vi "Excel_Title.vi"(7 "Report_Title":T1, 8 "error in (no error)":errorcluster, 10 "Report path in":path, 11 "Template path":path) -> (0 "error out":errorcluster, 2 "Report path out":path, 3 "report out":refnum<class "NI_report.lvclass">)   [LabVIEW 2015]
doc: "报表右上角的一大坨\n从编号到载荷时间"
uses:
  CustomControl/ReportTitle.ctl
  <vilib>/Utility/NIReport.llb/NI_report.lvclass
  <vilib>/addons/_office/NI_ReportGenerationToolkit.lvlib
  CustomControl/EnumReportTitle.ctl
panel:
  out "errorout":errorcluster
  in  "start(-1,-1) 2":cluster{"row":i32, "column":i32}
  in  "start(-1,-1)":cluster{"row":i32, "column":i32}
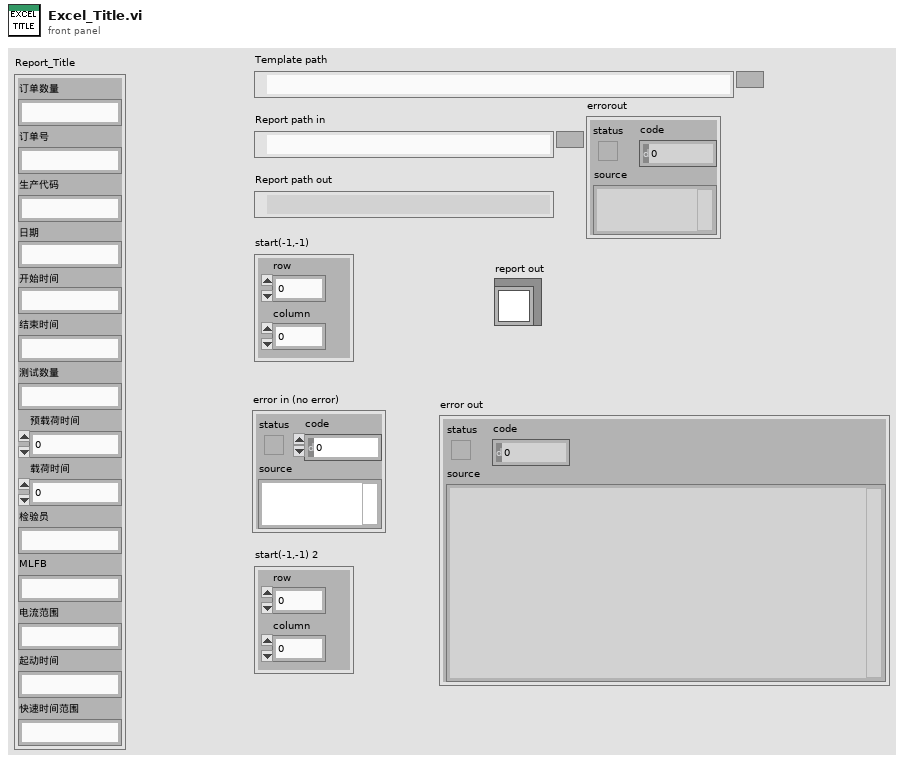
[diagram p1: front panel]
types:
  T1 = typedef "ReportTitle.ctl" = cluster{"订单数量":string, "订单号":string, "生产代码":string, "日期":string, "开始时间":string, "结束时间":string, "测试数量":string, "预载荷时间":i32, "载荷时间":i32, "检验员":string, "MLFB":string, "电流范围":string, "起动时间":string, "快速时间范围":string}
  T2 = enum16{"Standard Report", "HTML", "Word", "Excel"}
  T3 = enum16{"maximized", "minimized", "normal", "no change"}
  T4 = typedef "EnumReportTitle.ctl" = enum16{"CreatNewReport", "编号", "MLFB", "电流范围", "订单号", "订单数量", "测试日期", "检验员", "生产代码", "测试开始", "测试结束", "测试数量", "预载荷时间", "载荷时间", "起动时间", "快速动作范围", "CloseReport"}
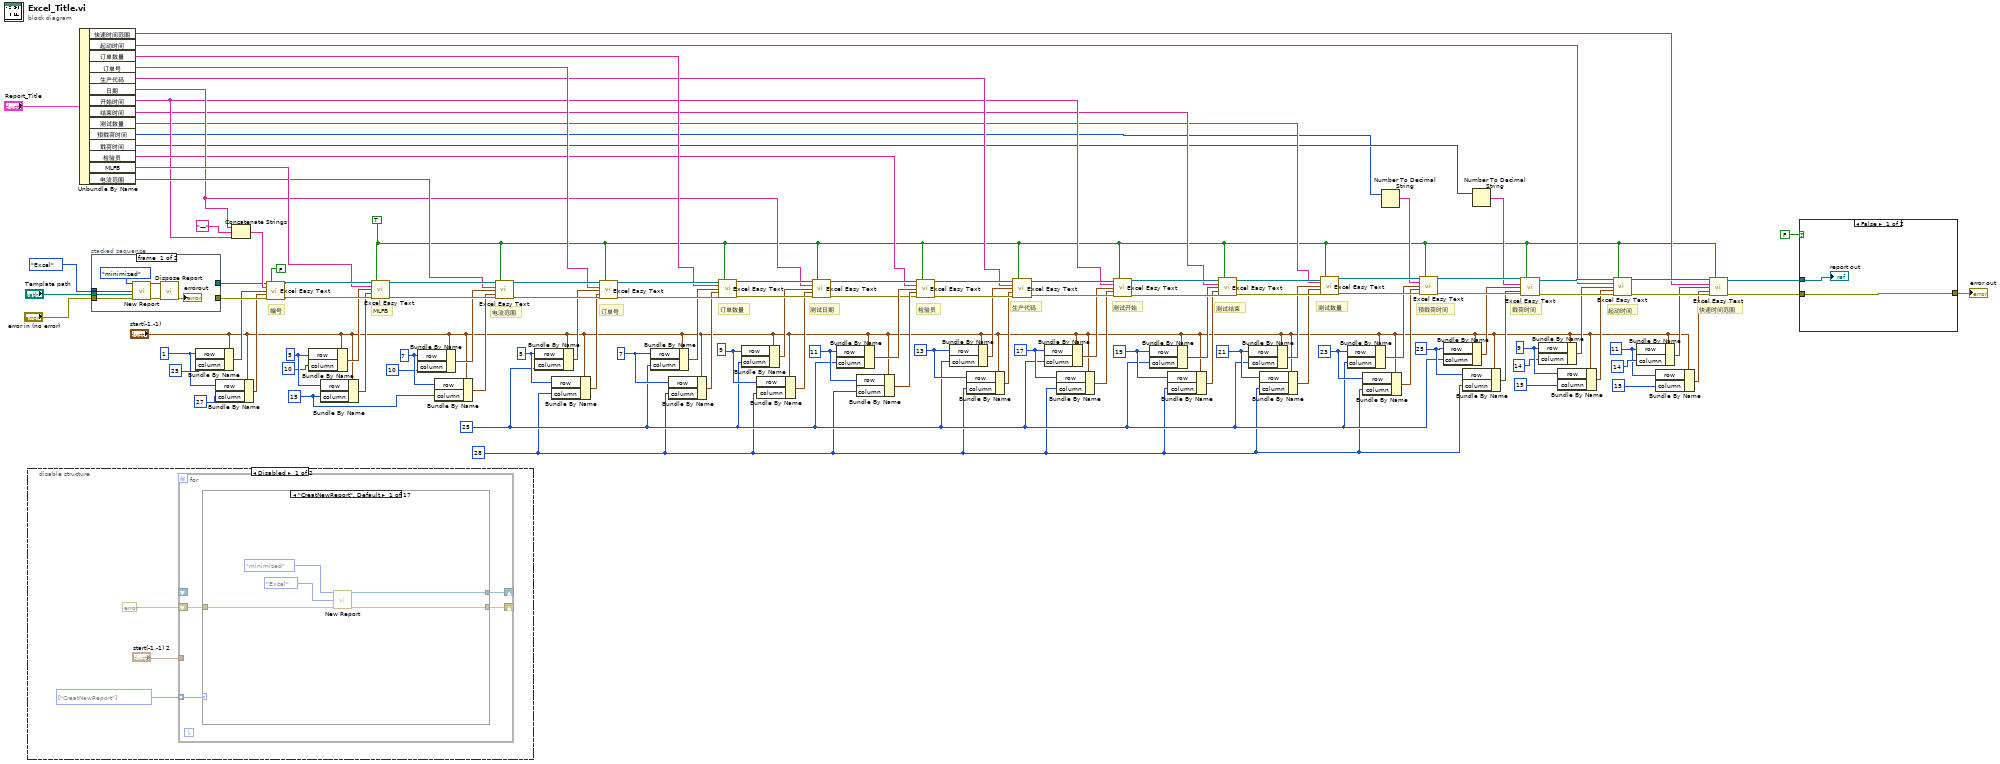
[diagram p0: block diagram]
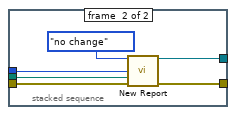
[diagram p2: hidden frame]
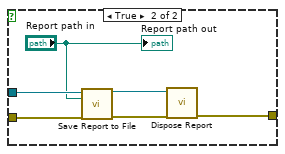
[diagram p20: hidden frame]
diagram:
  w5 = 11 ("row")
  w10 = 9 ("row")
  w43 = 25 ("row")
  w48 = 23 ("row")
  w53 = 21 ("row")
  w58 = 19 ("row")
  w63 = 17 ("row")
  w68 = 13 ("row")
  w75 = 11 ("row")
  w80 = 9 ("row")
  w41 = 28 ("column")
  w42 = 25 ("column")
  w83 = 7 ("column")
  w90 = 5 ("row")
  w103 = 7 ("row")
  w95 = 15 ("column")
  w99 = 5 ("row")
  w13 = TRUE ("border? (F)")
  w109 = 1 ("row")
  # "快速时间范围"
  # "起动时间"
  # "载荷时间"
  # "预载荷时间"
  # "测试数量"
  # "测试结束"
  # "测试开始"
  # "生产代码"
  # "检验员"
  # "测试日期"
  # "订单数量"
  # "订单号"
  # "编号"
  # "电流范围"
  # "MLFB"
  n1 = disable-structure shown="Disabled" {
    frame Disabled {
      w118 = T4[] [enum."CreatNewReport"] items=["CreatNewReport", "编号", "MLFB", "电流范围", "订单号", "订单数量", "测试日期", "检验员", "生产代码", "测试开始", "测试结束", "测试数量", "预载荷时间", "载荷时间", "起动时间", "快速动作范围", "CloseReport"]
      n2 = for {
        tunnel: w118 -> [w122] mode=indexing
        shift-right: [w120] -> _
        shift-left: errorcluster {"status"=FALSE, "code"=0, "source"=""} ("error out") -> [w121]
        shift-right: [w119] -> _
        shift-left: _ -> [_]
        tunnel: "start(-1,-1) 2" -> [_]
        n3 = case shown="\"CreatNewReport\", Default" w122 {
          tunnel: w121 -> [w125 _ _ _ _ _ _ _ _ _ _ _ _ _ _ _ _]
          tunnel: [w124 _ _ _ _ _ _ _ _ _ _ _ _ _ _ _ _] -> w120
          tunnel: [w123 _ _ _ _ _ _ _ _ _ _ _ _ _ _ _ _] -> w119
          frame "CreatNewReport", Default {
            n4 = call <vilib>:"New Report.vi"("window state (normal)"=T3."minimized", "report type"=T2."Excel", "error in (no error)"=w125) -> ("report out"=w123:refnum<class "NI_report.lvclass">, "error out"=w124:errorcluster)  [unwired: 11 in]
          }
          frame "编号" {
          }
          frame "MLFB" {
          }
          frame "电流范围" {
          }
          frame "订单号" {
          }
          frame "订单数量" {
          }
          frame "测试日期" {
          }
          frame "检验员" {
          }
          frame "生产代码" {
          }
          frame "测试开始" {
          }
          frame "测试结束" {
          }
          frame "测试数量" {
          }
          frame "预载荷时间" {
          }
          frame "载荷时间" {
          }
          frame "起动时间" {
          }
          frame "快速动作范围" {
          }
          frame "CloseReport" {
          }
        }
      }
    }
    frame Enabled {
    }
  }
  n5 = Unbundle By Name("Report_Title") -> ("快速时间范围"=w14:string, "起动时间"=w17:string, "订单数量"=w35:string, "订单号"=w36:string, "生产代码"=w32:string, "日期"=w34:string, "开始时间"=w31:string, "结束时间"=w30:string, "测试数量"=w29:string, "预载荷时间"=w25:i32, "载荷时间"=w27:i32, "检验员"=w33:string, "MLFB"=w38:string, "电流范围"=w37:string)
  n6 = stacked-sequence {
    tunnel: T2."Excel" ("report type") -> [w134 w138]
    tunnel: "Template path" -> [w133 w137]
    tunnel: "error in (no error)" -> [w132 w136]
    tunnel: [_ w140] -> w113
    tunnel: [_ w139] -> w114
    frame #0 {
      n7 = call <vilib>:"New Report.vi"("window state (normal)"=T3."minimized", "report type"=w134, "template (empty)"=w133, "error in (no error)"=w132) -> ("report out"=w130:refnum<class "NI_report.lvclass">, "error out"=w131:errorcluster)  [unwired: 10 in]
      n8 = call-dynamic "Dispose Report.vi"("report in"=w130, "error in (no error)"=w131) -> ("error out"=→"errorout":errorcluster)  [unwired: 13 in]
    }
    frame #1 {
      n9 = call <vilib>:"New Report.vi"("window state (normal)"=T3."no change", "report type"=w138, "template (empty)"=w137, "error in (no error)"=w136) -> ("report out"=w139:refnum<class "NI_report.lvclass">, "error out"=w140:errorcluster)  [unwired: 10 in]
    }
  }
  n10 = Bundle By Name(cluster="start(-1,-1)", "row"=w109, "column"=25) -> (w108:cluster{"row":i32, "column":i32})
  n11 = Bundle By Name(cluster="start(-1,-1)", "row"=w109, "column"=27) -> (w107:cluster{"row":i32, "column":i32})
  n12 = Concatenate Strings(w34, "—" ("string"), w31) -> (w115:string)
  n13 = call <vilib>:"Excel Easy Text.vi"("report in"=w114, "border? (F)"=FALSE, "text"=w115, "start (-1, -1)"=w108, "end (-1, -1)"=w107, "error in (no error)"=w113) -> ("report out"=w101:refnum<class "NI_report.lvclass">, "error out"=w100:errorcluster)  [unwired: 5 in, 3 out]
  n14 = Bundle By Name(cluster="start(-1,-1)", "row"=w99, "column"=10) -> (w97:cluster{"row":i32, "column":i32})
  n15 = Bundle By Name(cluster="start(-1,-1)", "row"=w99, "column"=w95) -> (w96:cluster{"row":i32, "column":i32})
  n16 = call <vilib>:"Excel Easy Text.vi"("report in"=w101, "border? (F)"=w13, "text"=w38, "start (-1, -1)"=w97, "end (-1, -1)"=w96, "error in (no error)"=w100) -> ("report out"=w105:refnum<class "NI_report.lvclass">, "error out"=w104:errorcluster)  [unwired: 5 in, 3 out]
  n17 = Bundle By Name(cluster="start(-1,-1)", "row"=w103, "column"=10) -> (w93:cluster{"row":i32, "column":i32})
  n18 = Bundle By Name(cluster="start(-1,-1)", "row"=w103, "column"=w95) -> (w94:cluster{"row":i32, "column":i32})
  n19 = call <vilib>:"Excel Easy Text.vi"("report in"=w105, "border? (F)"=w13, "text"=w37, "start (-1, -1)"=w93, "end (-1, -1)"=w94, "error in (no error)"=w104) -> ("report out"=w92:refnum<class "NI_report.lvclass">, "error out"=w91:errorcluster)  [unwired: 5 in, 3 out]
  n20 = Bundle By Name(cluster="start(-1,-1)", "row"=w90, "column"=w42) -> (w89:cluster{"row":i32, "column":i32})
  n21 = Bundle By Name(cluster="start(-1,-1)", "row"=w90, "column"=w41) -> (w88:cluster{"row":i32, "column":i32})
  n22 = call <vilib>:"Excel Easy Text.vi"("report in"=w92, "border? (F)"=w13, "text"=w36, "start (-1, -1)"=w89, "end (-1, -1)"=w88, "error in (no error)"=w91) -> ("report out"=w87:refnum<class "NI_report.lvclass">, "error out"=w86:errorcluster)  [unwired: 5 in, 3 out]
  n23 = Bundle By Name(cluster="start(-1,-1)", "row"=w83, "column"=w42) -> (w85:cluster{"row":i32, "column":i32})
  n24 = Bundle By Name(cluster="start(-1,-1)", "row"=w83, "column"=w41) -> (w84:cluster{"row":i32, "column":i32})
  n25 = call <vilib>:"Excel Easy Text.vi"("report in"=w87, "border? (F)"=w13, "text"=w35, "start (-1, -1)"=w85, "end (-1, -1)"=w84, "error in (no error)"=w86) -> ("report out"=w82:refnum<class "NI_report.lvclass">, "error out"=w81:errorcluster)  [unwired: 5 in, 3 out]
  n26 = Bundle By Name(cluster="start(-1,-1)", "row"=w80, "column"=w42) -> (w79:cluster{"row":i32, "column":i32})
  n27 = Bundle By Name(cluster="start(-1,-1)", "row"=w80, "column"=w41) -> (w78:cluster{"row":i32, "column":i32})
  n28 = call <vilib>:"Excel Easy Text.vi"("report in"=w82, "border? (F)"=w13, "text"=w34, "start (-1, -1)"=w79, "end (-1, -1)"=w78, "error in (no error)"=w81) -> ("report out"=w74:refnum<class "NI_report.lvclass">, "error out"=w73:errorcluster)  [unwired: 5 in, 3 out]
  n29 = Bundle By Name(cluster="start(-1,-1)", "row"=w75, "column"=w42) -> (w77:cluster{"row":i32, "column":i32})
  n30 = Bundle By Name(cluster="start(-1,-1)", "row"=w75, "column"=w41) -> (w76:cluster{"row":i32, "column":i32})
  n31 = call <vilib>:"Excel Easy Text.vi"("report in"=w74, "border? (F)"=w13, "text"=w33, "start (-1, -1)"=w77, "end (-1, -1)"=w76, "error in (no error)"=w73) -> ("report out"=w72:refnum<class "NI_report.lvclass">, "error out"=w71:errorcluster)  [unwired: 5 in, 3 out]
  n32 = Bundle By Name(cluster="start(-1,-1)", "row"=w68, "column"=w42) -> (w70:cluster{"row":i32, "column":i32})
  n33 = Bundle By Name(cluster="start(-1,-1)", "row"=w68, "column"=w41) -> (w69:cluster{"row":i32, "column":i32})
  n34 = call <vilib>:"Excel Easy Text.vi"("report in"=w72, "border? (F)"=w13, "text"=w32, "start (-1, -1)"=w70, "end (-1, -1)"=w69, "error in (no error)"=w71) -> ("report out"=w67:refnum<class "NI_report.lvclass">, "error out"=w66:errorcluster)  [unwired: 5 in, 3 out]
  n35 = Bundle By Name(cluster="start(-1,-1)", "row"=w63, "column"=w42) -> (w65:cluster{"row":i32, "column":i32})
  n36 = Bundle By Name(cluster="start(-1,-1)", "row"=w63, "column"=w41) -> (w64:cluster{"row":i32, "column":i32})
  n37 = call <vilib>:"Excel Easy Text.vi"("report in"=w67, "border? (F)"=w13, "text"=w31, "start (-1, -1)"=w65, "end (-1, -1)"=w64, "error in (no error)"=w66) -> ("report out"=w62:refnum<class "NI_report.lvclass">, "error out"=w61:errorcluster)  [unwired: 5 in, 3 out]
  n38 = Bundle By Name(cluster="start(-1,-1)", "row"=w58, "column"=w42) -> (w60:cluster{"row":i32, "column":i32})
  n39 = Bundle By Name(cluster="start(-1,-1)", "row"=w58, "column"=w41) -> (w59:cluster{"row":i32, "column":i32})
  n40 = call <vilib>:"Excel Easy Text.vi"("report in"=w62, "border? (F)"=w13, "text"=w30, "start (-1, -1)"=w60, "end (-1, -1)"=w59, "error in (no error)"=w61) -> ("report out"=w57:refnum<class "NI_report.lvclass">, "error out"=w56:errorcluster)  [unwired: 5 in, 3 out]
  n41 = Bundle By Name(cluster="start(-1,-1)", "row"=w53, "column"=w42) -> (w55:cluster{"row":i32, "column":i32})
  n42 = Bundle By Name(cluster="start(-1,-1)", "row"=w53, "column"=w41) -> (w54:cluster{"row":i32, "column":i32})
  n43 = call <vilib>:"Excel Easy Text.vi"("report in"=w57, "border? (F)"=w13, "text"=w29, "start (-1, -1)"=w55, "end (-1, -1)"=w54, "error in (no error)"=w56) -> ("report out"=w52:refnum<class "NI_report.lvclass">, "error out"=w51:errorcluster)  [unwired: 5 in, 3 out]
  n44 = Bundle By Name(cluster="start(-1,-1)", "row"=w48, "column"=w42) -> (w47:cluster{"row":i32, "column":i32})
  n45 = Bundle By Name(cluster="start(-1,-1)", "row"=w48, "column"=w41) -> (w46:cluster{"row":i32, "column":i32})
  n46 = Number To Decimal String(number=w25) -> (decimal integer string=w24:string)  [unwired: 1 in]
  n47 = call <vilib>:"Excel Easy Text.vi"("report in"=w52, "border? (F)"=w13, "text"=w24, "start (-1, -1)"=w47, "end (-1, -1)"=w46, "error in (no error)"=w51) -> ("report out"=w50:refnum<class "NI_report.lvclass">, "error out"=w49:errorcluster)  [unwired: 5 in, 3 out]
  n48 = Bundle By Name(cluster="start(-1,-1)", "row"=w43, "column"=w42) -> (w45:cluster{"row":i32, "column":i32})
  n49 = Bundle By Name(cluster="start(-1,-1)", "row"=w43, "column"=w41) -> (w44:cluster{"row":i32, "column":i32})
  n50 = Number To Decimal String(number=w27) -> (decimal integer string=w26:string)  [unwired: 1 in]
  n51 = call <vilib>:"Excel Easy Text.vi"("report in"=w50, "border? (F)"=w13, "text"=w26, "start (-1, -1)"=w45, "end (-1, -1)"=w44, "error in (no error)"=w49) -> ("report out"=w21:refnum<class "NI_report.lvclass">, "error out"=w20:errorcluster)  [unwired: 5 in, 3 out]
  n52 = Bundle By Name(cluster="start(-1,-1)", "row"=w10, "column"=14) -> (w12:cluster{"row":i32, "column":i32})
  n53 = Bundle By Name(cluster="start(-1,-1)", "row"=w10, "column"=15) -> (w11:cluster{"row":i32, "column":i32})
  n54 = call <vilib>:"Excel Easy Text.vi"("report in"=w21, "border? (F)"=w13, "text"=w17, "start (-1, -1)"=w12, "end (-1, -1)"=w11, "error in (no error)"=w20) -> ("report out"=w19:refnum<class "NI_report.lvclass">, "error out"=w18:errorcluster)  [unwired: 5 in, 3 out]
  n55 = Bundle By Name(cluster="start(-1,-1)", "row"=w5, "column"=14) -> (w3:cluster{"row":i32, "column":i32})
  n56 = Bundle By Name(cluster="start(-1,-1)", "row"=w5, "column"=15) -> (w4:cluster{"row":i32, "column":i32})
  n57 = call <vilib>:"Excel Easy Text.vi"("report in"=w19, "border? (F)"=w13, "text"=w14, "start (-1, -1)"=w3, "end (-1, -1)"=w4, "error in (no error)"=w18) -> ("report out"=w15:refnum<class "NI_report.lvclass">, "error out"=w16:errorcluster)  [unwired: 5 in, 3 out]
  n58 = case shown="False" FALSE {
    tunnel: w15 -> [w142 w146]
    tunnel: w16 -> [w141 w145]
    tunnel: [w141 w143] -> w23
    frame False {
      "report out" <- w142
    }
    frame True {
      n59 = call-dynamic "Save Report to File.vi"("report in"=w146, "report file path"="Report path in", "error in (no error)"=w145) -> ("report out"=w147:refnum<class "NI_report.lvclass">, "error out"=w148:errorcluster)  [unwired: 11 in]
      n60 = call-dynamic "Dispose Report.vi"("report in"=w147, "error in (no error)"=w148) -> ("error out"=w143:errorcluster)  [unwired: 13 in]
      "Report path out" <- "Report path in"
    }
  }
  "error out" <- w23
